vi "Change ports of s-parameters.vi"() -> ()   [LabVIEW 2020]
uses:
  <vilib>/addons/HF Network Analysis/Support VIs/Read SnP File (SnP).vi
  <vilib>/addons/HF Network Analysis/Support VIs/Read SnP File (S1P).vi
  <vilib>/addons/HF Network Analysis/NI_HFNetworkAnalysis.lvlib
panel:
  in  "Dummy S12, S21 data":cdb=1e-09+0.0i format="%#_13g"
  in  "Columns for s4p --> s2p":string="0,1,3,4"
  in  "Swap Ports (False)":bool
  out "resulting string":string
  in  "Columns for s3p --> s2p":string="0,1,3,4"
  in  "Column for sxp-->s1p":i32
  in  "To":enum16{"s1p", "s2p", "s3p", "s4p"}(ring)
  in  "From":enum16{"s1p", "s2p", "s3p", "s4p"}(ring)
  in  "Filename has to include:":string="s2p_DUT"
  in  "SnP File Path":path
  # "In    Out\n1      1\n2      1\n3      1\n1      2\n2      2\n3      2"
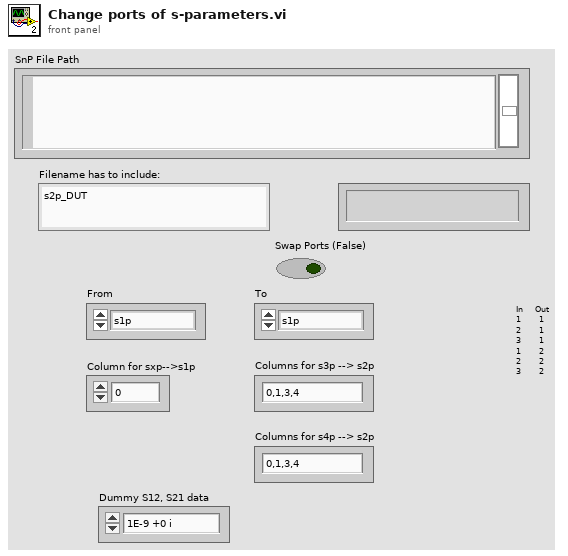
[diagram p1: front panel]
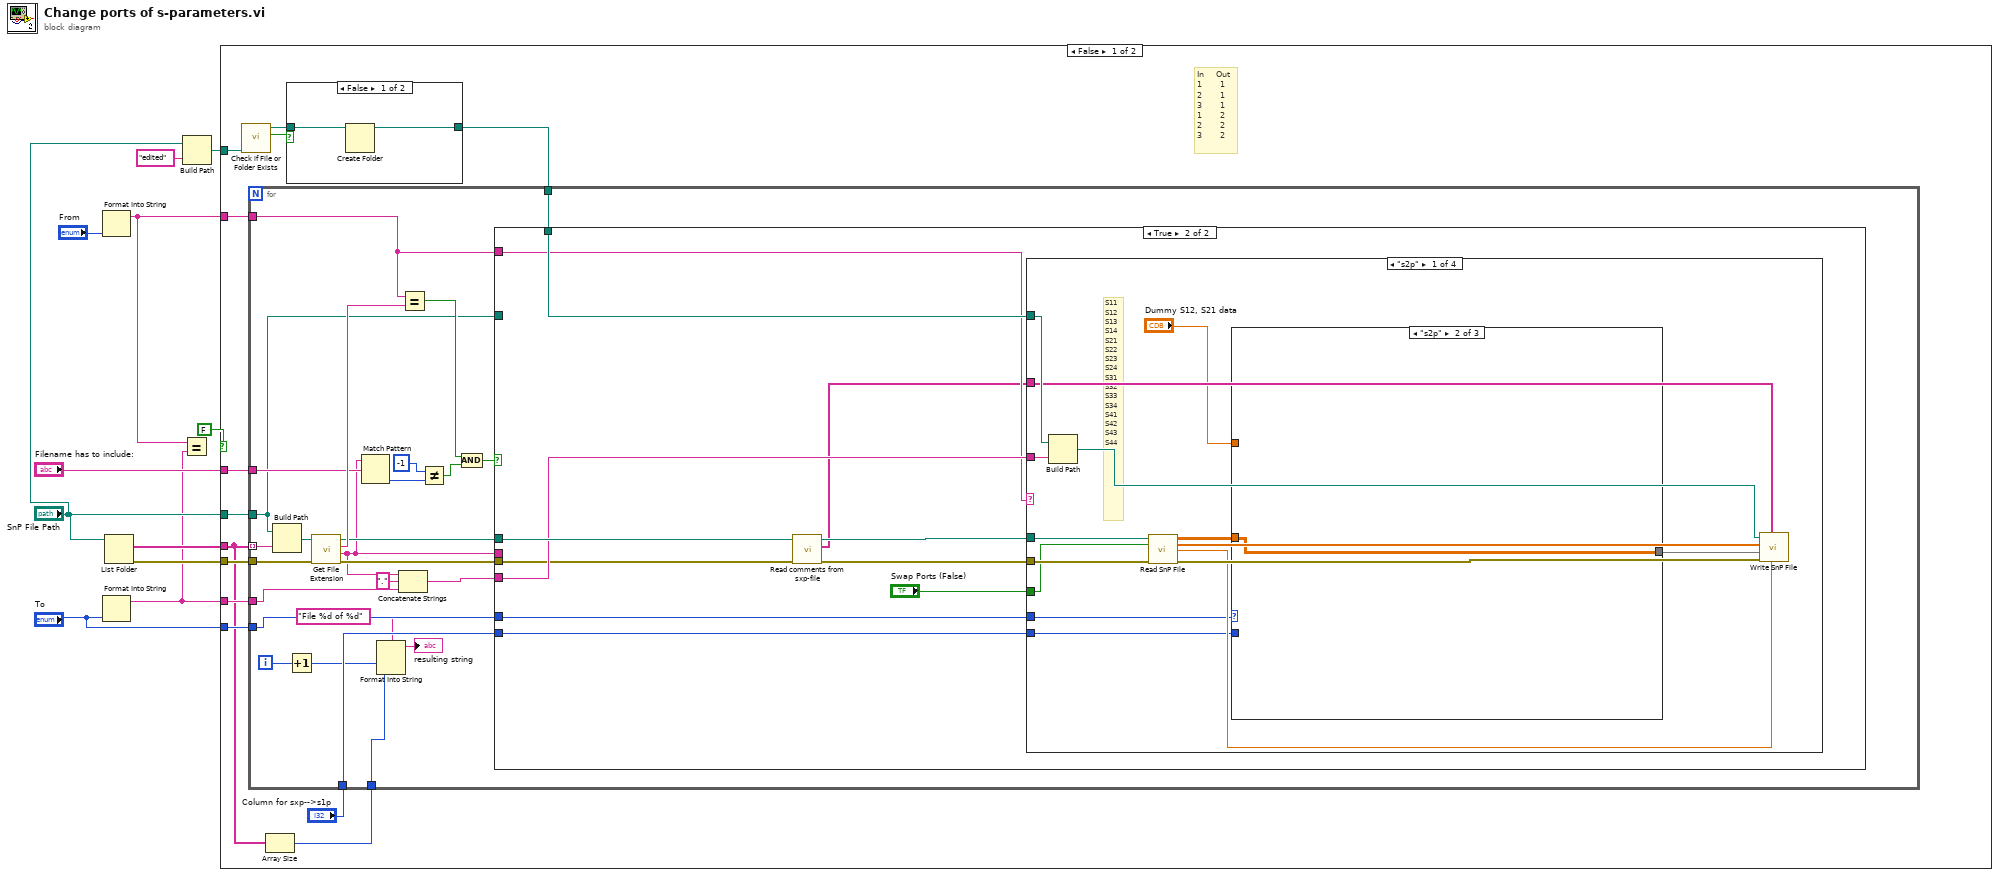
[diagram p0: block diagram]
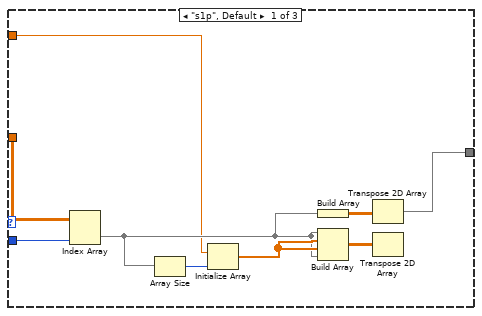
[diagram p4: hidden frame]
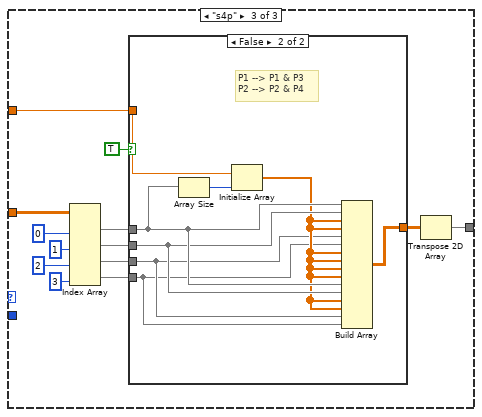
[diagram p5: hidden frame]
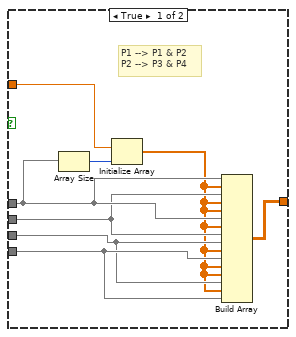
[diagram p6: hidden frame]
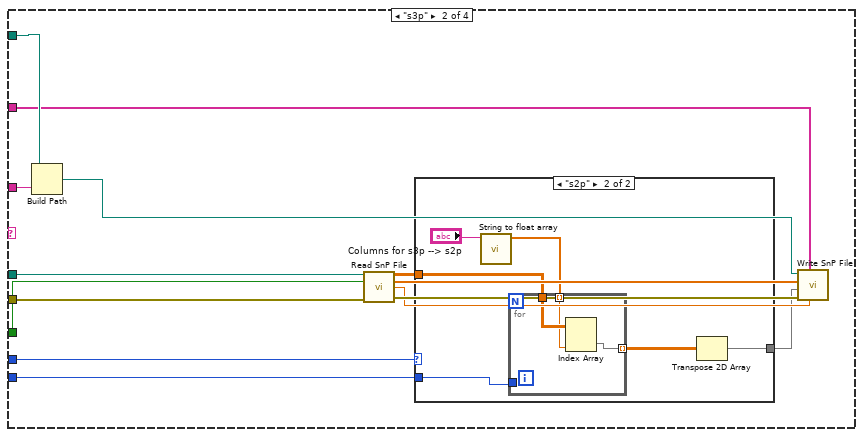
[diagram p7: hidden frame]
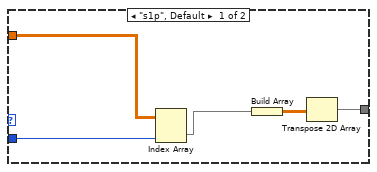
[diagram p8: hidden frame]
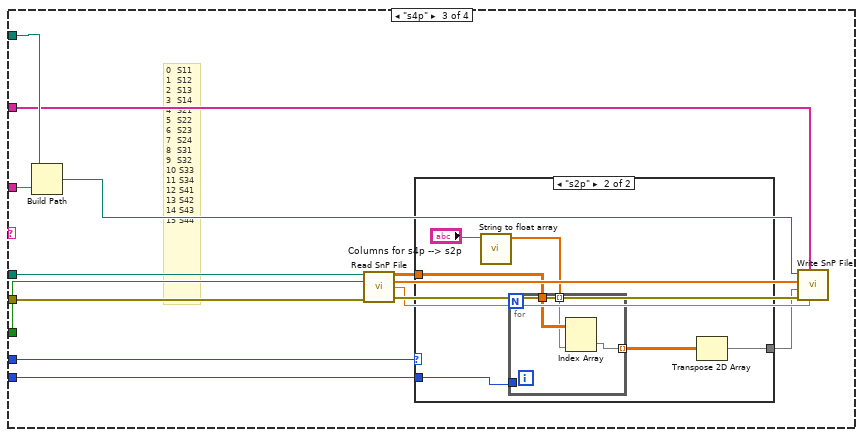
[diagram p9: hidden frame]
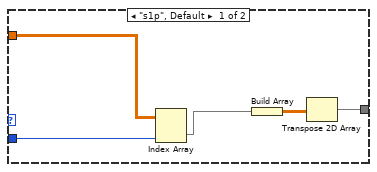
[diagram p10: hidden frame]
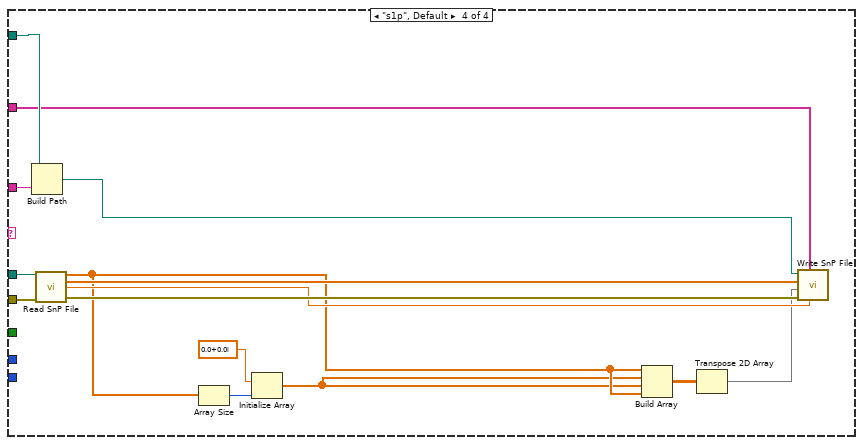
[diagram p11: hidden frame]
diagram:
  n1 = Format Into String("From") -> (resulting string=w4:string)  [unwired: 3 in, 1 out]
  n2 = Format Into String("To") -> (resulting string=w3:string)  [unwired: 3 in, 1 out]
  n3 = List Folder(path="SnP File Path") -> (filenames=w11:string[], error out=w9:errorcluster)  [unwired: 3 in, 2 out]
  n4 = Equal?(x=w4, y=w3) -> ()  [unwired: 1 out]
  n5 = Build Path(base path="SnP File Path", name or relative path="edited") -> (appended path=w6:path)
  n6 = case shown="False" FALSE {
    tunnel: w11 -> [w13 _]
    tunnel: "Filename has to include:" -> [w24 _]
    tunnel: w9 -> [w23 _]
    tunnel: "SnP File Path" -> [w22 _]
    tunnel: w6 -> [w21 _]
    tunnel: w4 -> [w17 _]
    tunnel: w3 -> [w16 _]
    tunnel: "To" -> [w14 _]
    frame False {
      # "In    Out\n1      1\n2      1\n3      1\n1      2\n2      2\n3      2"
      n7 = call <vilib>:"Check if File or Folder Exists.vi"("path"=w21) -> ("file or folder exists?"=w19:bool, "dup path"=w20:path)  [unwired: 8 in, 1 out]
      n8 = Array Size(array=w13) -> (size(s)=w12:i32)
      n9 = case shown="False" w19 {
        tunnel: w20 -> [w26 w27]
        tunnel: [w25 w27] -> w18
        frame False {
          n10 = Create Folder(path (use dialog)=w26) -> (created path=w25:path)  [unwired: 2 in, 2 out]
        }
        frame True {
        }
      }
      n11 = for {
        tunnel: w13 -> [w49] mode=indexing
        tunnel: w22 -> [w40]
        tunnel: w24 -> [w48]
        tunnel: w23 -> [w47]
        tunnel: w18 -> [w39]
        tunnel: w17 -> [w36]
        tunnel: w16 -> [w38]
        tunnel: "Column for sxp-->s1p" -> [w34]
        tunnel: w14 -> [w33]
        tunnel: w12 -> [w29]
        i -> [w31]
        n12 = Build Path(base path=w40, name or relative path=w49) -> (appended path=w52:path)
        n13 = Increment(x=w31) -> (x+1=w30:i32)
        n14 = call <vilib>:"Get File Extension.vi"("error in (no error)"=w47, "file"=w52) -> ("error out"=w46:errorcluster, "filename without extension"=w44:string, "lowercase file extension"=w50:string, "dup file"=w45:path)  [unwired: 5 in, 1 out]
        n15 = Match Pattern(string=w44, regular expression=w48) -> (offset past match=w51:i32)  [unwired: 1 in, 3 out]
        n16 = Format Into String(format string="File %d of %d", w30, w29) -> (resulting string=→"resulting string":string)  [unwired: 2 in, 1 out]
        n17 = Concatenate Strings(w44, "." ("string"), w38) -> (w37:string)
        n18 = Equal?(x=w36, y=w50) -> (x = y?=w42:bool)
        n19 = Not Equal?(x=-1, y=w51) -> (x != y?=w43:bool)
        n20 = And(x=w42, y=w43) -> (x .and. y?=w41:bool)
        n21 = case shown="True" w41 {
          tunnel: w46 -> [_ w58]
          tunnel: w45 -> [_ w64]
          tunnel: w44 -> [_ _]
          tunnel: w40 -> [_ _]
          tunnel: w39 -> [_ w63]
          tunnel: w37 -> [_ w62]
          tunnel: w36 -> [_ w61]
          tunnel: w34 -> [_ w60]
          tunnel: w33 -> [_ w59]
          frame False {
          }
          frame True {
            n22 = call "Read comments from sxp-file.vi"("error in (no error)"=w58, "file path"=w64) -> ("error out"=w56:errorcluster, "Comment lines"=w55:string[], "file path out"=w57:path)  [unwired: 7 in]
            n23 = case shown="\"s2p\"" w61 {
              tunnel: w56 -> [w70 w132 w160 w189]
              tunnel: w57 -> [w71 w131 w159 w188]
              tunnel: w63 -> [w75 w126 w154 w183]
              tunnel: w62 -> [w74 w124 w152 w177]
              tunnel: w60 -> [w73 w122 w150 _]
              tunnel: w59 -> [w66 w121 w149 _]
              tunnel: w55 -> [w72 w120 w148 w175]
              tunnel: "Swap Ports (False)" -> [w69 w119 w147 _]
              frame "s2p" {
                # "S11\nS12\nS13\nS14\nS21\nS22\nS23\nS24\nS31\nS32\nS33\nS34\nS41\nS42\nS43\nS44"
                n24 = Build Path(base path=w75, name or relative path=w74) -> (appended path=w76:path)
                n25 = call-poly <vilib>:"Read SnP File.vi"("SnP File Path"=w71, "Swap Ports (False)"=w69, "Error In"=w70) -> ("S-parameters"=w68:cdb[][], "Frequencies (Hz)"=w79:dbl[], "Z0 (Ohm)"=w77:cdb, "Error Out"=w78:errorcluster)  [unwired: 9 in]
                n26 = case shown="\"s2p\"" w66 {
                  tunnel: w73 -> [w83 _ _]
                  tunnel: w68 -> [w82 w89 w100]
                  tunnel: [w81 w89 w101] -> w67
                  tunnel: "Dummy S12, S21 data" -> [w80 _ w90]
                  frame "s1p", Default {
                    n27 = Index Array(array=w82, index (col)=w83) -> (element=w85:cdb[])  [unwired: 1 in]
                    n28 = Array Size(array=w85) -> (size(s)=w88:i32)
                    n29 = Initialize Array(w80, w88) -> (w87:cdb[])
                    n30 = Build Array(w85) -> (w84:cdb[][])
                    n31 = Build Array(w85, w87, w87, w85) -> (w86:cdb[][])
                    n32 = Transpose 2D Array(2D array=w84) -> (transposed array=w81:cdb[][])
                    n33 = Transpose 2D Array(2D array=w86) -> ()  [unwired: 1 out]
                  }
                  frame "s2p" {
                  }
                  frame "s4p" {
                    n34 = Index Array(array=w100, index (col) #1=0 ("disabled index (col)"), index (col) #2=1 ("index (col)"), index (col) #3=2 ("index (col)"), index (col) #4=3 ("index (col)")) -> (element #1=w99:cdb[], element #2=w98:cdb[], element #3=w97:cdb[], element #4=w96:cdb[])  [unwired: 4 in]
                    n35 = case shown="False" TRUE {
                      tunnel: [w109 w117] -> w102
                      tunnel: w99 -> [w108 w116]
                      tunnel: w98 -> [w107 w115]
                      tunnel: w97 -> [w105 w113]
                      tunnel: w96 -> [w106 w112]
                      tunnel: w90 -> [w103 w111]
                      frame True {
                        # "P1 --> P1 & P2\nP2 --> P3 & P4"
                        n36 = Array Size(array=w108) -> (size(s)=w110:i32)
                        n37 = Initialize Array(w103, w110) -> (w104:cdb[])
                        n38 = Build Array(w108, w104, w107, w104, w104, w108, w104, w107, w105, w104, w106, w104, w104, w105, w104, w106) -> (w109:cdb[][])
                      }
                      frame False {
                        # "P1 --> P1 & P3\nP2 --> P2 & P4"
                        n39 = Array Size(array=w116) -> (size(s)=w118:i32)
                        n40 = Initialize Array(w111, w118) -> (w114:cdb[])
                        n41 = Build Array(w116, w115, w114, w114, w113, w112, w114, w114, w114, w114, w116, w115, w114, w114, w113, w112) -> (w117:cdb[][])
                      }
                    }
                    n42 = Transpose 2D Array(2D array=w102) -> (transposed array=w101:cdb[][])
                  }
                }
                n43 = call <vilib>:"Write SnP File.vi"("Z0 (50 Ohm)"=w77, "Comments"=w72, "error in (no error)"=w78, "S-parameters"=w67, "Frequencies (Hz)"=w79, "SnP File Path"=w76) -> ()  [unwired: 5 in, 1 out]
              }
              frame "s3p" {
                n44 = Build Path(base path=w126, name or relative path=w124) -> (appended path=w127:path)
                n45 = call-poly <vilib>:"Read SnP File.vi"("SnP File Path"=w131, "Swap Ports (False)"=w119, "Error In"=w132) -> ("S-parameters"=w125:cdb[][], "Frequencies (Hz)"=w130:dbl[], "Z0 (Ohm)"=w128:cdb, "Error Out"=w129:errorcluster)  [unwired: 9 in]
                n46 = case shown="\"s2p\"" w121 {
                  tunnel: w125 -> [w137 w143]
                  tunnel: [w134 w138] -> w123
                  tunnel: w122 -> [w133 w142]
                  frame "s1p", Default {
                    n47 = Index Array(array=w137, index (col)=w133) -> (element=w136:cdb[])  [unwired: 1 in]
                    n48 = Build Array(w136) -> (w135:cdb[][])
                    n49 = Transpose 2D Array(2D array=w135) -> (transposed array=w134:cdb[][])
                  }
                  frame "s2p" {
                    n50 = call "String to float array.vi"("String"="Columns for s3p --> s2p") -> ("Array - Numeric"=w140:dbl[])  [unwired: 9 in, 1 out]
                    n51 = for {
                      tunnel: w143 -> [w146]
                      tunnel: [w144] -> w139 mode=indexing
                      tunnel: w142 -> [_]
                      tunnel: w140 -> [w145] mode=indexing
                      n52 = Index Array(array=w146, index (col)=w145) -> (element=w144:cdb[])  [unwired: 1 in]
                    }
                    n53 = Transpose 2D Array(2D array=w139) -> (transposed array=w138:cdb[][])
                  }
                }
                n54 = call <vilib>:"Write SnP File.vi"("Z0 (50 Ohm)"=w128, "Comments"=w120, "error in (no error)"=w129, "S-parameters"=w123, "Frequencies (Hz)"=w130, "SnP File Path"=w127) -> ()  [unwired: 5 in, 1 out]
              }
              frame "s4p" {
                # "0 \tS11\n1 \tS12\n2 \tS13\n3 \tS14\n4 \tS21\n5 \tS22\n6 \tS23\n7 \tS24\n8 \tS31\n9 \tS32\n10\tS33\n11\tS34\n12\tS41\n13\tS42\n14\tS43\n15\tS44"
                n55 = Build Path(base path=w154, name or relative path=w152) -> (appended path=w155:path)
                n56 = call-poly <vilib>:"Read SnP File.vi"("SnP File Path"=w159, "Swap Ports (False)"=w147, "Error In"=w160) -> ("S-parameters"=w153:cdb[][], "Frequencies (Hz)"=w158:dbl[], "Z0 (Ohm)"=w156:cdb, "Error Out"=w157:errorcluster)  [unwired: 9 in]
                n57 = case shown="\"s2p\"" w149 {
                  tunnel: w153 -> [w165 w171]
                  tunnel: [w162 w166] -> w151
                  tunnel: w150 -> [w161 w170]
                  frame "s1p", Default {
                    n58 = Index Array(array=w165, index (col)=w161) -> (element=w164:cdb[])  [unwired: 1 in]
                    n59 = Build Array(w164) -> (w163:cdb[][])
                    n60 = Transpose 2D Array(2D array=w163) -> (transposed array=w162:cdb[][])
                  }
                  frame "s2p" {
                    n61 = call "String to float array.vi"("String"="Columns for s4p --> s2p") -> ("Array - Numeric"=w168:dbl[])  [unwired: 9 in, 1 out]
                    n62 = for {
                      tunnel: w171 -> [w174]
                      tunnel: [w172] -> w167 mode=indexing
                      tunnel: w170 -> [_]
                      tunnel: w168 -> [w173] mode=indexing
                      n63 = Index Array(array=w174, index (col)=w173) -> (element=w172:cdb[])  [unwired: 1 in]
                    }
                    n64 = Transpose 2D Array(2D array=w167) -> (transposed array=w166:cdb[][])
                  }
                }
                n65 = call <vilib>:"Write SnP File.vi"("Z0 (50 Ohm)"=w156, "Comments"=w148, "error in (no error)"=w157, "S-parameters"=w151, "Frequencies (Hz)"=w158, "SnP File Path"=w155) -> ()  [unwired: 5 in, 1 out]
              }
              frame "s1p", Default {
                n66 = Build Path(base path=w183, name or relative path=w177) -> (appended path=w184:path)
                n67 = call-poly <vilib>:"Read SnP File.vi"("S1P File Path"=w188, "Error In"=w189) -> ("S-parameters"=w180:cdb[], "Frequencies (Hz)"=w187:dbl[], "Z0 (Ohm)"=w185:cdb, "Error Out"=w186:errorcluster)  [unwired: 10 in]
                n68 = Array Size(array=w180) -> (size(s)=w182:i32)
                n69 = Initialize Array(cdb 0.0+0.0i ("Numeric Control"), w182) -> (w179:cdb[])
                n70 = Build Array(w180, w179, w179, w180) -> (w178:cdb[][])
                n71 = Transpose 2D Array(2D array=w178) -> (transposed array=w176:cdb[][])
                n72 = call <vilib>:"Write SnP File.vi"("Z0 (50 Ohm)"=w185, "Comments"=w175, "error in (no error)"=w186, "S-parameters"=w176, "Frequencies (Hz)"=w187, "SnP File Path"=w184) -> ()  [unwired: 5 in, 1 out]
              }
            }
          }
        }
      }
    }
    frame True {
    }
  }
